vi "UT_004_LV to TMOL.vi"() -> ()   [LabVIEW 2017]
uses:
  <vilib>/addons/_JKI Toolkits/Caraya/classes/Assert/Assert True.vi
  <vilib>/addons/_JKI Toolkits/Caraya/classes/Test/Test.lvclass
  lib/TOML.lvlib
  <vilib>/addons/_JKI Toolkits/Caraya/classes/Assert/Assert.lvclass
panel:
  out "toml String 3":string
  out "toml String 2":string
  out "toml String":string
  out "error out 3":errorcluster
  out "error out":errorcluster
  out "error out 2":errorcluster
  in  "data 3":string[][](array[string])=[["a", "b"], ["d", "e"], ["g", "h"]]
  in  "data 2":string[][](array[string])=[["a", "b", "c"], ["d", "e", "f"]]
  in  "data":string[][](array[string])=[["a", "b", "c"], ["d", "e", "f"], ["g", "h", "i"]]
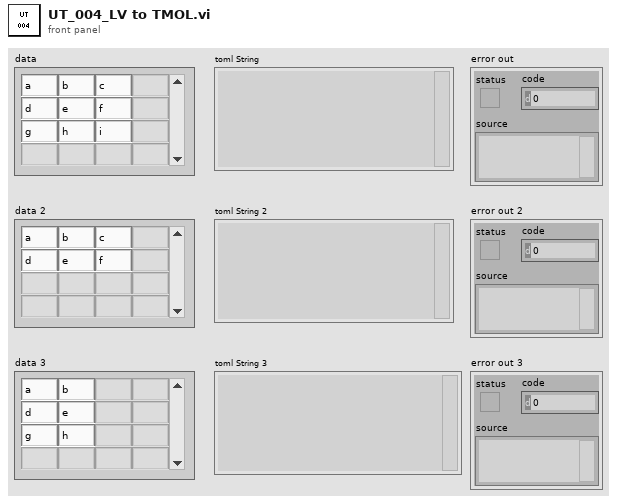
[diagram p1: front panel]
types:
  T1 = typedef "TOML.lvlib/TOML Value.ctl" = cluster{"type":enum16{"Table", "Array", "String", "Integer", "Float", "Boolean", "Offset Date-Time", "Local Date-Time", "Local Date", "Local Time"}, "value":variant}
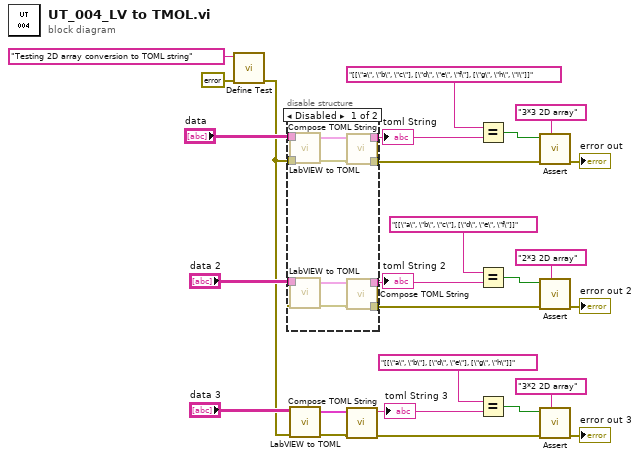
[diagram p0: block diagram]
diagram:
  n1 = call <vilib>:"Define Test.vi"("error in (no error)"=errorcluster {"status"=FALSE, "code"=0, "source"=""}, "Label (VI Title)"="Testing 2D array conversion to TOML string") -> ("error out"=w9:errorcluster)  [unwired: 9 in]
  n2 = disable-structure shown="Disabled" {
    disable-tunnel: "data 2" -> [w37 _]
    disable-tunnel: [w34 _] -> w22
    disable-tunnel: [w33 _] -> w19
    disable-tunnel: [w32 _] -> w18
    disable-tunnel: "data" -> [w29 _]
    disable-tunnel: w9 -> [w28 _]
    disable-tunnel: [w27 _] -> w3
    frame Disabled {
      n3 = call "LabVIEW to TOML.vi"("error in (no error)"=w28, "LV Value"=w29) -> ("error out"=w30:errorcluster, "TOML Value"=w31:T1)  [unwired: 8 in]
      n4 = call "LabVIEW to TOML.vi"("error in (no error)"=w28, "LV Value"=w37) -> ("error out"=w36:errorcluster, "TOML Value"=w35:T1)  [unwired: 8 in]
      n5 = call "Compose TOML String.vi"("error in (no error)"=w30, "Value"=w31) -> ("error out"=w32:errorcluster, "String"=w33:string)  [unwired: 8 in]
      n6 = call "Compose TOML String.vi"("error in (no error)"=w36, "Value"=w35) -> ("error out"=w34:errorcluster, "String"=w27:string)  [unwired: 8 in]
    }
    frame Enabled {
    }
  }
  "toml String" <- w19
  "toml String 2" <- w3
  n7 = call "LabVIEW to TOML.vi"("error in (no error)"=w9, "LV Value"="data 3") -> ("error out"=w11:errorcluster, "TOML Value"=w12:T1)  [unwired: 8 in]
  n8 = call "Compose TOML String.vi"("error in (no error)"=w11, "Value"=w12) -> ("error out"=w14:errorcluster, "String"=w2:string)  [unwired: 8 in]
  "toml String 3" <- w2
  n9 = Equal?(x="[[\"a\", \"b\", \"c\"], [\"d\", \"e\", \"f\"], [\"g\", \"h\", \"i\"]]", y=w19) -> (x = y?=w1:bool)
  n10 = Equal?(x="[[\"a\", \"b\", \"c\"], [\"d\", \"e\", \"f\"]]", y=w3) -> (x = y?=w21:bool)
  n11 = Equal?(x="[[\"a\", \"b\"], [\"d\", \"e\"], [\"g\", \"h\"]]", y=w2) -> (x = y?=w15:bool)
  n12 = call-poly <vilib>:"Assert.vi"("Label"="3*3 2D array" ("Label (VI Title)"), "error in (no error)"=w18, "True?"=w1) -> ("error out"=→"error out":errorcluster)  [unwired: 8 in]
  n13 = call-poly <vilib>:"Assert.vi"("Label"="2*3 2D array" ("Label (VI Title)"), "error in (no error)"=w22, "True?"=w21) -> ("error out"=→"error out 2":errorcluster)  [unwired: 8 in]
  n14 = call-poly <vilib>:"Assert.vi"("Label"="3*2 2D array" ("Label (VI Title)"), "error in (no error)"=w14, "True?"=w15) -> ("error out"=→"error out 3":errorcluster)  [unwired: 8 in]
